vi "Get All Refs (SubVI).vi"(0 "Current VI Path":path, 11 "Error IN":errorcluster) -> (4 "Control Refs":cluster{"Label Name":string, "Ref":refnum<vi>}[](array[cluster]), 15 "Error OUT":errorcluster)   [LabVIEW 2012]
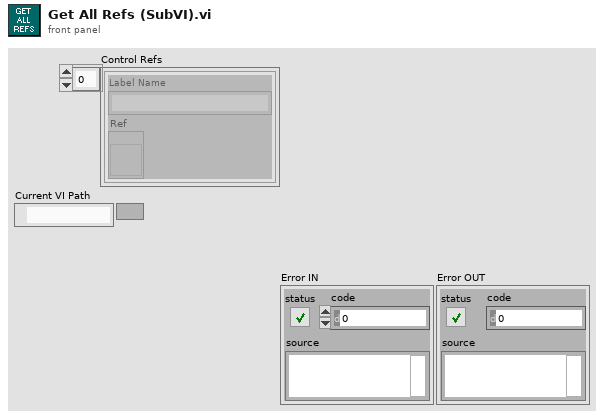
[diagram p1: front panel]
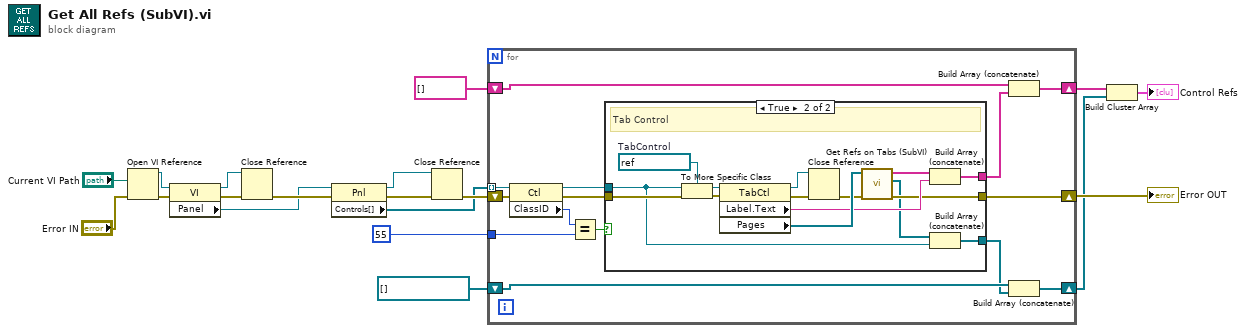
[diagram p0: block diagram]
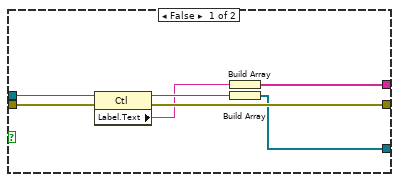
[diagram p2: hidden frame]
diagram:
  n1 = Open VI Reference(vi path="Current VI Path", error in (no error)="Error IN") -> (vi reference=w2:refnum<vi>, error out=w5:errorcluster)  [unwired: 4 in]
  n2 = property class="VI"(reference=w2, error in=w5) -> (reference out=w15:refnum<vi>, error out=w16:errorcluster, "Panel"=w6:refnum<vi>)
  n3 = Close Reference(reference=w15, error in (no error)=w16) -> (error out=w17:errorcluster)
  n4 = property class="Pnl"(reference=w6, error in=w17) -> (reference out=w12:refnum<vi>, error out=w13:errorcluster, "Controls[]"=w3:refnum<vi>[])
  n5 = Close Reference(reference=w12, error in (no error)=w13) -> (error out=w14:errorcluster)
  n6 = for {
    tunnel: w3 -> [w31] mode=indexing
    shift-right: [w33] -> w9
    shift-left: refnum<vi>[] [] -> [w32]
    shift-right: [w23] -> w10
    shift-left: w14 -> [w30]
    shift-right: [w28] -> w8
    shift-left: string[] [] -> [w29]
    tunnel: u32 55 -> [w22]
    n7 = property class="Ctl"(reference=w31, error in=w30) -> (reference out=w26:refnum<vi>, error out=w24:errorcluster, "ClassID"=w27:u32)
    n8 = Equal?(x=w27, y=w22) -> (x = y?=w25:bool)
    n9 = case shown="True" w25 {
      tunnel: w26 -> [w40 w46]
      tunnel: [w34 w44] -> w20
      tunnel: w24 -> [w39 w54]
      tunnel: [w38 w48] -> w23
      tunnel: [w36 w45] -> w21
      frame False {
        n10 = property class="Ctl"(reference=w40, error in=w39) -> (reference out=w37:refnum<vi>, error out=w38:errorcluster, "Label.Text"=w35:string)
        n11 = Build Array(w35) -> (w34:string[])
        n12 = Build Array(w37) -> (w36:refnum<vi>[])
      }
      frame True {
        w52 = refnum<vi> refnum  # TabControl
        # "Tab Control"
        n13 = To More Specific Class(target class=w52, reference=w46, error in=w54) -> (specific class reference=w55:refnum<vi>, error out=w53:errorcluster)
        n14 = property class="TabCtl"(reference=w55, error in=w53) -> (reference out=w43:refnum<vi>, error out=w42:errorcluster, "Label.Text"=w50:string, "Pages"=w51:refnum<vi>[])
        n15 = Close Reference(reference=w43, error in (no error)=w42) -> (error out=w41:errorcluster)
        n16 = call "Get Refs on Tabs (SubVI).vi"("error in (no error)"=w41, "Pages"=w51) -> ("error out"=w48:errorcluster, "Refs"=w47:refnum<vi>[], "Labels"=w49:string[])  [unwired: 7 in]
        n17 = Build Array (concatenate)(w49, w50) -> (w44:string[])
        n18 = Build Array (concatenate)(w47, w46) -> (w45:refnum<vi>[])
      }
    }
    n19 = Build Array (concatenate)(w29, w20) -> (w28:string[])
    n20 = Build Array (concatenate)(w32, w21) -> (w33:refnum<vi>[])
  }
  "Error OUT" <- w10
  n21 = Build Cluster Array(w8, w9) -> (→"Control Refs":cluster{string, refnum<vi>}[])
